vi "Update Parameters.vi"(8 "error in (no error)":errorcluster, 11 "Triangle in":refnum<class "Triangle.lvclass">) -> (0 "error out":errorcluster, 3 "Triangle out":refnum<class "Triangle.lvclass">)   [LabVIEW 2014]
uses:
  Triangle.lvclass
  Waveform/Waveform.lvclass
panel:
  in  "Amplitude":dbl
  in  "Offset":dbl
  in  "Frequency":dbl
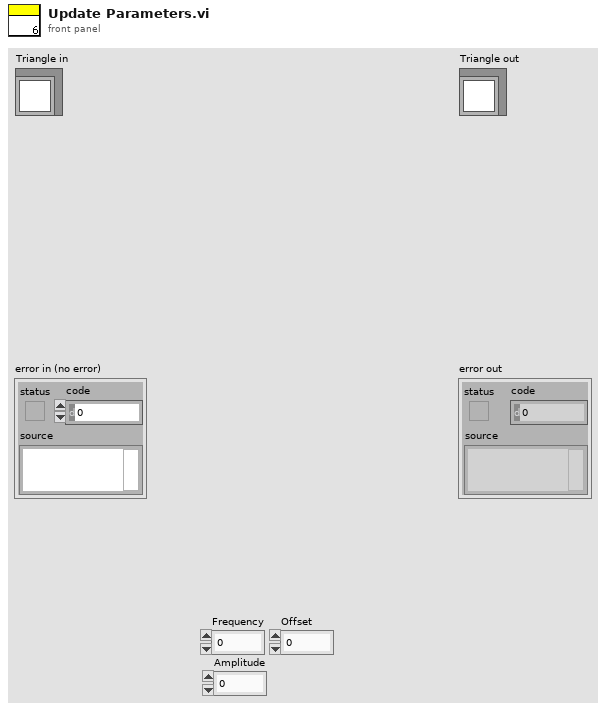
[diagram p1: front panel]
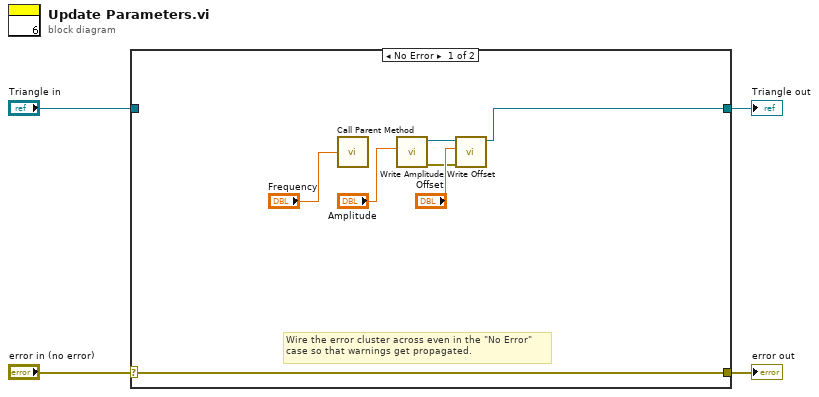
[diagram p0: block diagram]
diagram:
  n1 = case shown="No Error" "error in (no error)" {
    selector: "error in (no error)" -> [w14 w16]
    tunnel: [w14 w16] -> w3
    tunnel: [w5 w15] -> w1
    tunnel: "Triangle in" -> [w6 w15]
    frame No Error {
      # "Wire the error cluster across even in the \"No Error\"\ncase so that warnings get propagated."
      n2 = call-parent "Call Parent Method"("Frequency") -> ()
      n3 = call-dynamic "Write Amplitude.vi"("Amplitude"="Amplitude") -> ("error out"=w10:errorcluster, "Waveform out"=w8:refnum<class "Triangle.lvclass">, "error in (no error)"=w11:errorcluster, "Waveform in"=w9:refnum<class "Triangle.lvclass">)  [unwired: 7 in]
      n4 = call "Write Offset.vi"("error in (no error)"=w10, "Offset"="Offset", "Waveform in"=w8) -> ("Waveform out"=w5:refnum<class "Triangle.lvclass">)  [unwired: 7 in, 1 out]
    }
    frame Error {
    }
  }
  "error out" <- w3
  "Triangle out" <- w1
